vi "Day 1 - Historian Hysteria.vi"() -> ()   [LabVIEW 2020, in "AoC 2024.lvlib"]
uses:
  AoC 2024.lvlib
  <userlib>/_OpenG.lib/array/array.llb/Search 1D Array (I32)__ogtk.vi
  <userlib>/_OpenG.lib/array/array.llb/openg_array.lvlib
panel:
  out "Puzzle Part-2 Answer":string
  out "Puzzle Answer":string
  in  "Puzzle Input":string="3   4\n4   3\n2   5\n1   3\n3   9\n3   3"
  # "Enter the Puzzle Input and run the VI"
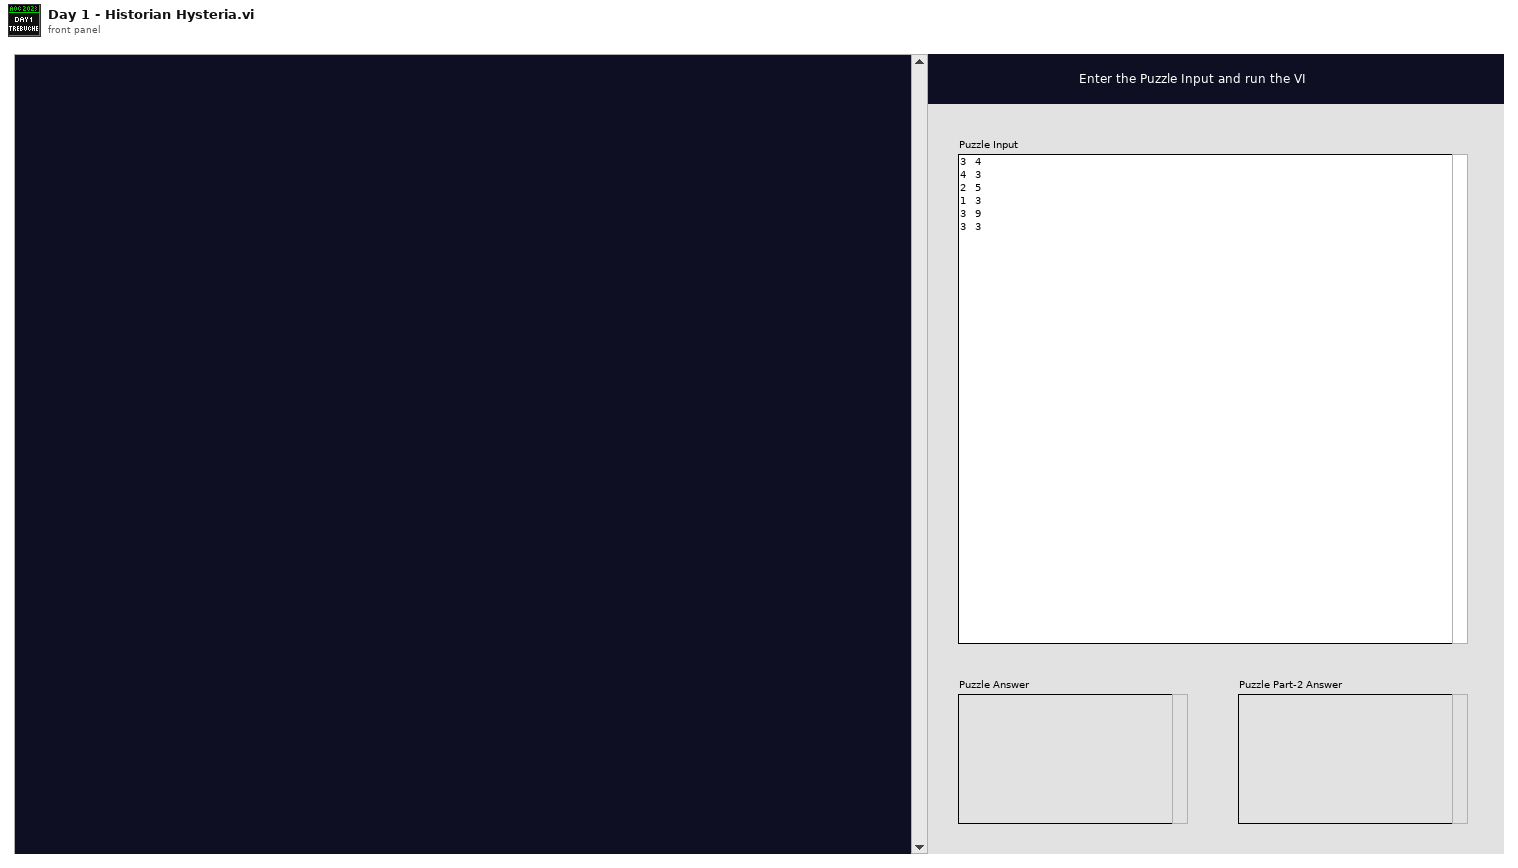
[diagram p1: front panel]
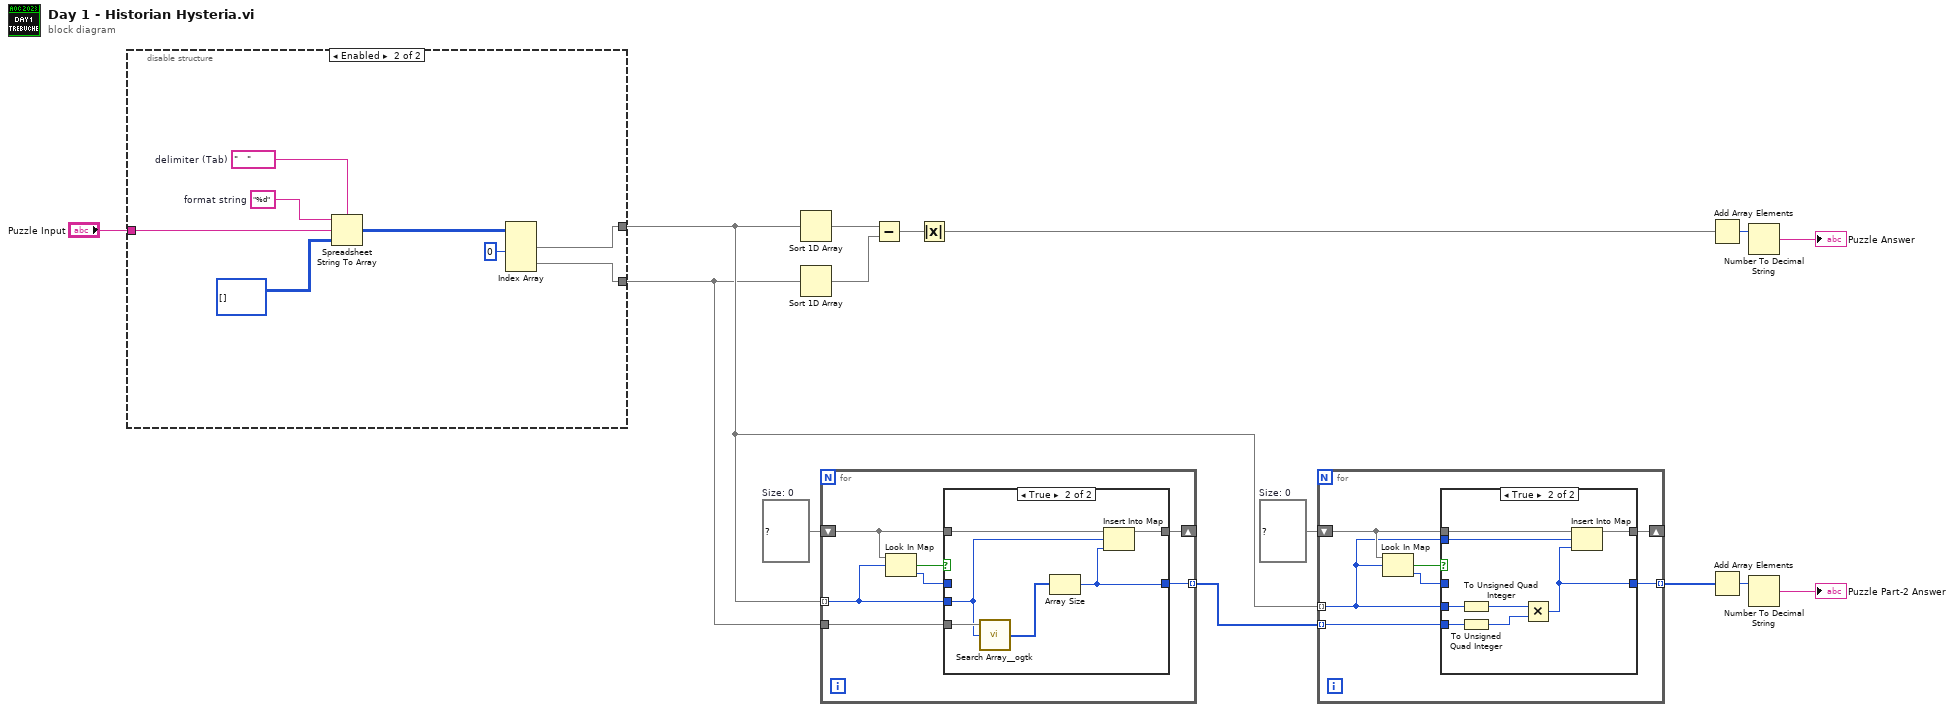
[diagram p0: block diagram]
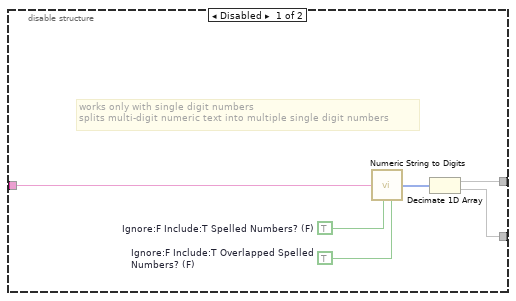
[diagram p2: hidden frame]
diagram:
  w7 = map{i32, u64} {}  # Size: 0
  w8 = map{i32, i32} {}  # Size: 0
  n1 = disable-structure shown="Enabled" {
    disable-tunnel: "Puzzle Input" -> [w21 w29]
    disable-tunnel: [w17 w24] -> w2
    disable-tunnel: [w16 w23] -> w1
    frame Disabled {
      w19 = TRUE  # Ignore:F Include:T Overlapped Spelled Numbers? (F)
      w20 = TRUE  # Ignore:F Include:T Spelled Numbers? (F)
      # "works only with single digit numbers\nsplits multi-digit numeric text into multiple single digit numbers"
      n2 = call "Numeric String to Digits.vi"("Numeric String"=w21, "Ignore:F Include:T Spelled Numbers? (F)"=w20, "Ignore:F Include:T Overlapped Spelled Numbers? (F)"=w19) -> ("Digits"=w18:i32[])
      n3 = Decimate 1D Array(w18) -> (w17:i32[], w16:i32[])
    }
    frame Enabled {
      w27 = "   "  # delimiter (Tab)
      w28 = "%d"  # format string
      n4 = Spreadsheet String To Array(delimiter (Tab)=w27, format string=w28, spreadsheet string=w29, array type (2D Dbl)=i32[][] []) -> (array=w25:i32[][])
      n5 = Index Array(array=w25, index (col) #1=0 ("disabled index (col)")) -> (element #1=w24:i32[], element #2=w23:i32[])  [unwired: 3 in]
    }
  }
  n6 = Sort 1D Array(array=w2) -> (sorted array=w9:i32[])
  n7 = Sort 1D Array(array=w1) -> (sorted array=w10:i32[])
  n8 = for {
    tunnel: w2 -> [w30] mode=indexing
    tunnel: w1 -> [w31]
    shift-right: [w36] -> _
    shift-left: w8 -> [w35]
    tunnel: [w32] -> w6 mode=indexing
    n9 = Look In Map(map=w35, key=w30) -> (key not found?=w34:bool, value=w33:i32)  [unwired: 1 in]
    n10 = case shown="True" w34 {
      tunnel: [w37 w44] -> w36
      tunnel: w35 -> [w37 w43]
      tunnel: w30 -> [_ w41]
      tunnel: w33 -> [w38 _]
      tunnel: [w38 w39] -> w32
      tunnel: w31 -> [_ w42]
      frame False {
      }
      frame True {
        n11 = call-poly <userlib>:"Search Array__ogtk.vi"("Array"=w42, "Element Data"=w41) -> ("Indices of Elements"=w40:i32[])  [unwired: 7 in]
        n12 = Array Size(array=w40) -> (size(s)=w39:i32)
        n13 = Insert Into Map(map in=w43, key=w41, value=w39) -> (map out=w44:map{i32, i32})  [unwired: 2 out]
      }
    }
  }
  n14 = Subtract(x=w9, y=w10) -> (x-y=w12:i32[])
  n15 = Absolute Value(x=w12) -> (abs(x)=w11:i32[])
  n16 = for {
    tunnel: w2 -> [w45] mode=indexing
    tunnel: w6 -> [w46] mode=indexing
    shift-right: [w51] -> _
    shift-left: w7 -> [w50]
    tunnel: [w47] -> w4 mode=indexing
    n17 = Look In Map(map=w50, key=w45) -> (key not found?=w49:bool, value=w48:u64)  [unwired: 1 in]
    n18 = case shown="True" w49 {
      tunnel: [w52 w61] -> w51
      tunnel: w50 -> [w52 w60]
      tunnel: w45 -> [_ w59]
      tunnel: w48 -> [w53 _]
      tunnel: [w53 w56] -> w47
      tunnel: w46 -> [_ w57]
      tunnel: w45 -> [_ w58]
      frame False {
      }
      frame True {
        n19 = To Unsigned Quad Integer(1:w58) -> (0:w55:u64)
        n20 = To Unsigned Quad Integer(1:w57) -> (0:w54:u64)
        n21 = Multiply(x=w55, y=w54) -> (x*y=w56:u64)
        n22 = Insert Into Map(map in=w60, key=w59, value=w56) -> (map out=w61:map{i32, u64})  [unwired: 2 out]
      }
    }
  }
  n23 = Add Array Elements(numeric array=w11) -> (sum=w13:i32)
  n24 = Add Array Elements(numeric array=w4) -> (sum=w5:u64)
  n25 = Number To Decimal String(number=w13) -> (decimal integer string=→"Puzzle Answer":string)  [unwired: 1 in]
  n26 = Number To Decimal String(number=w5) -> (decimal integer string=→"Puzzle Part-2 Answer":string)  [unwired: 1 in]
